vi "onDestroy.vi"(8 "error in (no error)":errorcluster, 11 "Pump.Simulated":refnum<class "Pump.Simulated.lvclass">) -> (0 "error out":errorcluster, 3 "Pump.Simulated out":refnum<class "Pump.Simulated.lvclass">)   [LabVIEW 2014, in "Pump.Simulated.lvclass"]
doc: "JKI State Machine Objects (SMO) 1.4.0.57\nJKI - JKI\nCopyright (c) 2018, JKI"
uses:
  Pump.Simulated.lvclass
  Pump.Simulated.lvclass/Pump.Simulated.ctl
  Pump class/Pump.lvclass
panel:
  # "For instructions on how to use the JKI State Machine Objects, examples and video tutorials, visit:\nhttp://jki.net/state-machine-objects/\n\nJKI State Machine Objects™\nhttp://jki.net/state-machine-objects/\nCopyright (C) 2005-2015, JKI <info@jki.net>\nALL RIGHTS RESERVED"
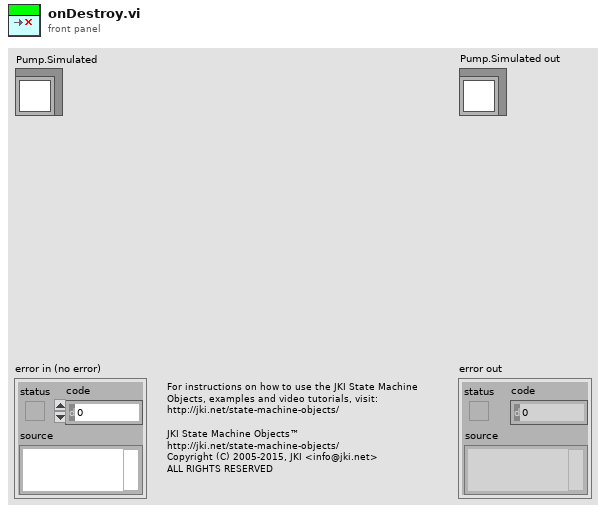
[diagram p1: front panel]
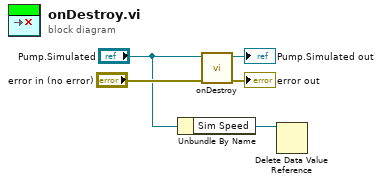
[diagram p0: block diagram]
diagram:
  n1 = Unbundle By Name("Pump.Simulated") -> ("Sim Speed"=w1:refnum<data-value>)
  n2 = call-parent "onDestroy.vi"("error in (no error)"="error in (no error)", "Pump"="Pump.Simulated") -> ("error out"=→"error out":errorcluster, "Pump out"=→"Pump.Simulated out":refnum<class "Pump.Simulated.lvclass">)  [unwired: 8 in]
  n3 = Delete Data Value Reference(data value reference=w1) -> ()  [unwired: 1 in, 2 out]
